vi "BTS 1.vi"() -> ()   [LabVIEW 2024]
panel:
  out "indicador 1":dbl[](array[numeric])
  in  "Boolean 2":bool
  out "String":string="essa é uma string"
  out "Boolean":bool=TRUE
  in  "VALOR N":dbl
  out "Slide 2":dbl(slide) scale=0.0..200.0
  in  "suga 2 - 1":dbl
  in  "jin 2 - 0":dbl
  out "BTS":i32
  in  "jungkook 1 - 1":dbl
  in  "jimin 1 - 0":dbl
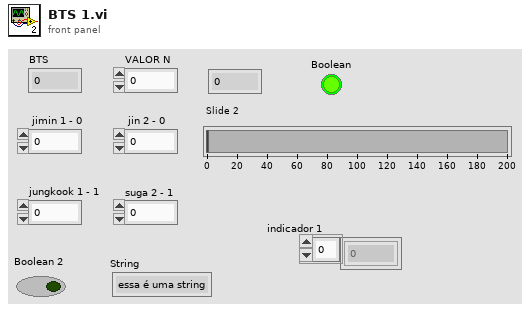
[diagram p1: front panel]
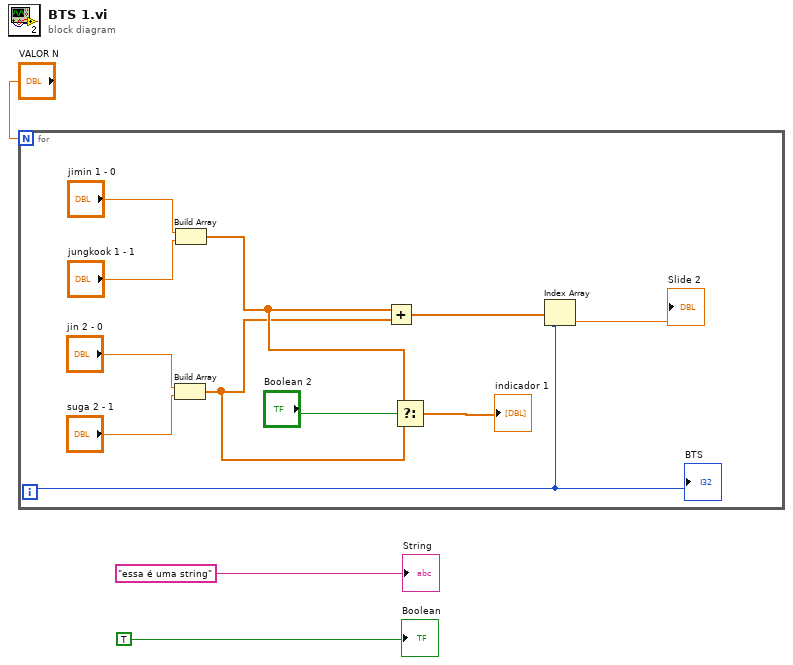
[diagram p0: block diagram]
diagram:
  n1 = for {
    N: "VALOR N" -> [_]
    i -> [w9]
    n2 = Build Array("jin 2 - 0", "suga 2 - 1") -> (w6:dbl[])
    n3 = Build Array("jimin 1 - 0", "jungkook 1 - 1") -> (w7:dbl[])
    n4 = Add(x=w7, y=w6) -> (x+y=w10:dbl[])
    n5 = Select(t=w7, s="Boolean 2", f=w6) -> (s? t:f=→"indicador 1":dbl[])
    n6 = Index Array(array=w10, index=w9) -> (element=→"Slide 2":dbl)
    "BTS" <- w9
  }
  "Boolean" <- TRUE
  "String" <- "essa é uma string"
